vi "白下黑下.vi"(11 "下棋步数":i32) -> (2 "Enum":enum16{"黑棋下", "白棋下"}(ring)=enum."白棋下", 8 "下棋步数":i32, 15 "黑白棋一共的下棋步数":i32)   [LabVIEW 2018]
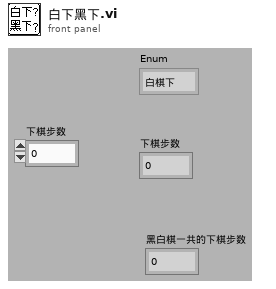
[diagram p1: front panel]
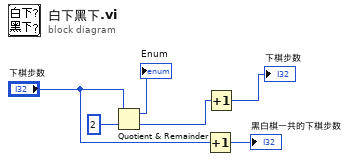
[diagram p0: block diagram]
diagram:
  n1 = Quotient & Remainder(x="下棋步数", y=2) -> (x-y*floor(x/y)=→"Enum":i32, floor(x/y)=w2:i32)
  n2 = Increment(x="下棋步数") -> (x+1=→"黑白棋一共的下棋步数":i32)
  n3 = Increment(x=w2) -> (x+1=→"下棋步数":i32)
